vi "SetActualPosition.vi"(0 "handle in":i32, 1 "UnitAddress(0)":u16, 2 "MotNr(0)":u8, 5 "error in":errorcluster, 7 "ActualPosition(0)":i32) -> (14 "handle out":i32, 19 "error out":errorcluster)   [LabVIEW 2014, in "Sixpack - Driver.lvlib"]
doc: "ACHTUNG: Wird ein Referenzschalter verwendet, kann die Benutzung dieses Befehls zu einer Referenzfahrt mit anschließender Zurücksetzung des Positionszählers führen. Der Befehl verändert den Wert des internen Positionszählers.\n\nCMD $27\nMotorNr (0...5)\nPosAkt: neue aktuelle Position"
uses:
  Sixpack - Driver.lvlib
  DLL/PackDLL.dll
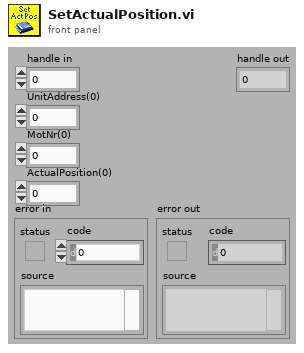
[diagram p1: front panel]
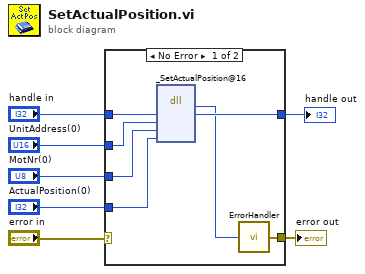
[diagram p0: block diagram]
diagram:
  n1 = case shown="No Error" "error in" {
    selector: "error in" -> [_ w15]
    tunnel: "handle in" -> [w14 w16]
    tunnel: [w13 w16] -> w6
    tunnel: "UnitAddress(0)" -> [w12 _]
    tunnel: "MotNr(0)" -> [w11 _]
    tunnel: "ActualPosition(0)" -> [w10 _]
    tunnel: [w9 w15] -> w2
    frame No Error {
      n2 = dll-call lib="D:/CS-Source/LV2014/GPL/instr.lib/SixPack/PackDLL/DLL/PackDLL.dll" fn="_SetActualPosition@16" label="SetActualPosition"("HANDLE"=w14, "UnitAddress"=w12, "MotNr"=w11, "ActualPosition"=w10) -> ("BOOLEAN"=w8:i8, "HANDLE"=w13:i32)  [unwired: 6 in, 2 out]
      n3 = call "ErrorHandler.vi"("BOOLEAN"=w8) -> ("error out"=w9:errorcluster)
    }
    frame Error {
    }
  }
  "handle out" <- w6
  "error out" <- w2
